vi "Filter Inbound Message.vi"(10 "Message":refnum<class "Message.lvclass">, 11 "Pub Sub Message Channel in":refnum<class "Pub Sub Message Channel.lvclass">) -> (2 "Drop Message":bool, 3 "Pub Sub Message Channel out":refnum<class "Pub Sub Message Channel.lvclass">)   [LabVIEW 2020, in "Actor Pub Sub Channels.lvlib" / "Pub Sub Message Channel.lvclass"]
uses:
  Pub Sub Message Channel.lvclass
  <vilib>/ActorFramework/Message/Message.lvclass
  Pub Sub Message Channel.lvclass/Pub Sub Message Channel.ctl
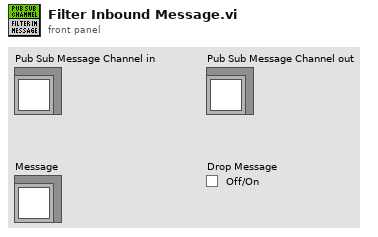
[diagram p1: front panel]
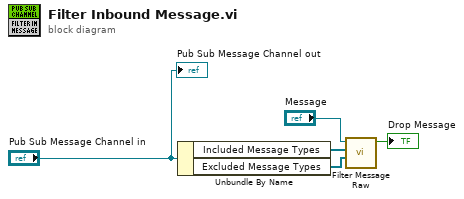
[diagram p0: block diagram]
diagram:
  n1 = Unbundle By Name("Pub Sub Message Channel in") -> ("Included Message Types"=w2:refnum<class "Message.lvclass">[], "Excluded Message Types"=w3:refnum<class "Message.lvclass">[])
  n2 = call "Filter Message Raw.vi"("Excluded Message Types"=w3, "Included Message Types"=w2, "Message in"="Message") -> ("Checkbox"=→"Drop Message":bool)  [unwired: 8 in]
  "Pub Sub Message Channel out" <- "Pub Sub Message Channel in"
